vi "L298N_Controller.vi"(8 "Error In":errorcluster caption="Entrée d'erreur", 10 "Action_Moteur":T9, 11 "Cluster":T1) -> (0 "Error Out":errorcluster caption="Sortie d'erreur")   [LabVIEW 2019]
uses:
  L298N_Action_Enum.ctl
  L298N_Ref_Type.ctl
  <vilib>/myRIO/Instrument Drivers/Onboard IO/DIO/typedefs/DIO Reference.ctl
  <vilib>/myRIO/Common/Instrument Driver Framework/Utilities/typedefs/myRIO Generic Hardware Reference.ctl
  <vilib>/myRIO/Common/Instrument Driver Framework/Utilities/typedefs/Hardware Version Enum.ctl
  <vilib>/myRIO/Common/Instrument Driver Framework/Utilities/typedefs/myRIO v1.0 Reference.ctl
  <vilib>/myRIO/Common/Instrument Driver Framework/Utilities/typedefs/Generic FPGA Reference.ctl
  <vilib>/myRIO/Common/Instrument Driver Framework/myRIO v1.0/DIO/typedefs/DIO Channels List.ctl
  <vilib>/myRIO/Common/Instrument Driver Framework/myRIO v1.0/DIO/typedefs/DIO Channels Enum.ctl
  <vilib>/Utility/error.llb/Error Cluster From Error Code.vi
  <vilib>/myRIO/Common/Instrument Driver Framework/myRIO v1.0/DIO/vis/myRIO v1.0 Write DIO.vi
  <vilib>/myRIO/Instrument Drivers/Onboard IO/DIO/DIO.lvlib
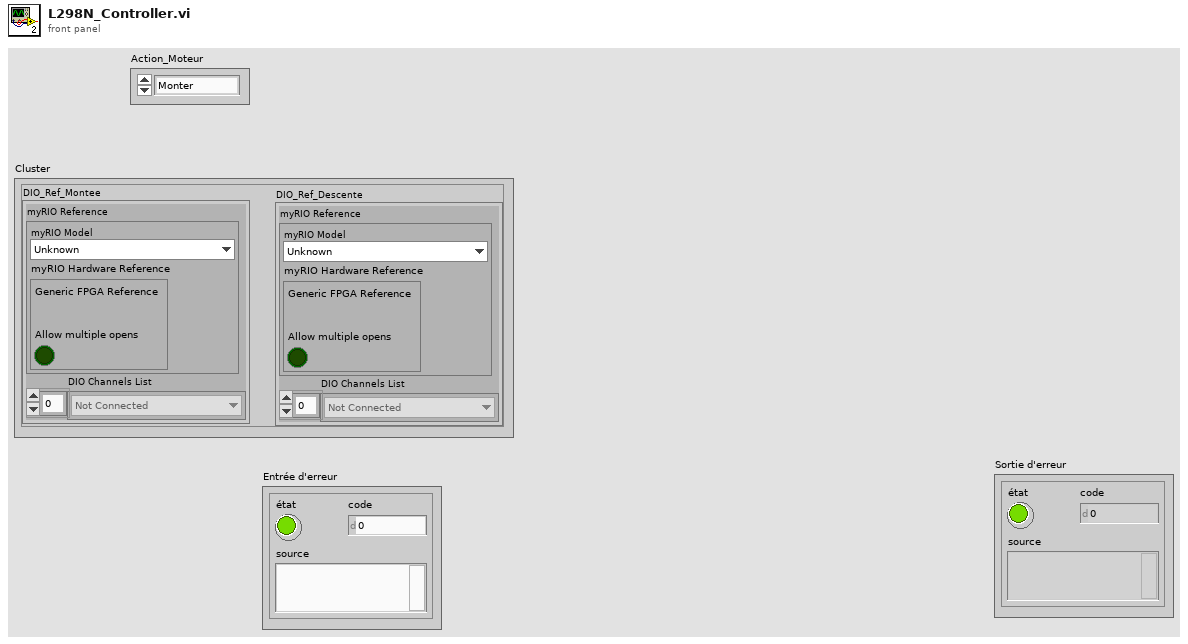
[diagram p1: front panel]
types:
  T1 = typedef "L298N_Ref_Type.ctl" = cluster{"DIO_Ref_Montee":T2, "DIO_Ref_Descente":T2}
  T2 = typedef "DIO.lvlib/DIO Reference.ctl" = cluster{"myRIO Reference":T3, "DIO Channels List":T7}
  T3 = typedef "myRIO Generic Hardware Reference.ctl" = cluster{"myRIO Model":T4, "myRIO Hardware Reference":T5}
  T4 = typedef "Hardware Version Enum.ctl" = enum16{"Unknown", "myRIO-1900", "myRIO-1950", "roboRIO", "NI ELVIS RIO CM", "ELVIS III"}
  T5 = typedef "myRIO v1.0 Reference.ctl" = cluster{"Generic FPGA Reference":T6, "Allow multiple opens":bool}
  T6 = typedef "Generic FPGA Reference.ctl" = refnum<k20>
  T7 = typedef "DIO Channels List.ctl" = T8[]
  T8 = typedef "DIO Channels Enum.ctl" = enum16{"Not Connected", "C/DIO0", "C/DIO1", "C/DIO2", "C/DIO3", "C/DIO4", "C/DIO5", "C/DIO6", "C/DIO7", "A/DIO0", "A/DIO1", "A/DIO2", "A/DIO3", "A/DIO4", "A/DIO5", "A/DIO6", "A/DIO7", "A/DIO8", "A/DIO9", "A/DIO10", "A/DIO11", "A/DIO12", "A/DIO13", "A/DIO14", "A/DIO15", "A/DIO16", "A/DIO17", "A/DIO18", "A/DIO19", "B/DIO0", "B/DIO1", "B/DIO2", "B/DIO3", "B/DIO4", "B/DIO5", "B/DIO6", "B/DIO7", "B/DIO8", "B/DIO9", "B/DIO10", "B/DIO11", "B/DIO12", "B/DIO13", "B/DIO14", "B/DIO15", "B/DIO16", "B/DIO17", "B/DIO18", "B/DIO19", "LED0", "LED1", "LED2", "LED3", "Button0", "DIO/DIO0", "DIO/DIO1", "DIO/DIO2", "DIO/DIO3", "DIO/DIO4", "DIO/DIO5", "DIO/DIO6", "DIO/DIO7", "DIO/DIO8", "DIO/DIO9", "SPI/CS0", "SPI/CS1", "SPI/CS2", "SPI/CS3", "LED RADIO (Green)", "LED RADIO (Red)", "LED COMM (Green)", "LED COMM (Red)", "LED MODE (Green)", "LED MODE (Red)"}
  T9 = typedef "L298N_Action_Enum.ctl" = enum16{"Monter", "Descendre", "Arreter"}
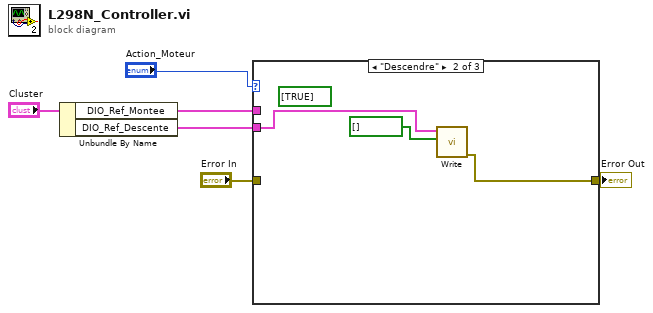
[diagram p0: block diagram]
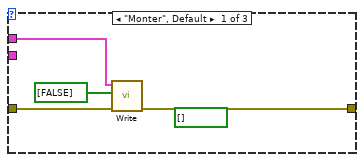
[diagram p2: hidden frame]
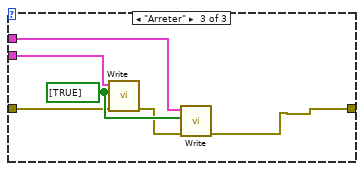
[diagram p3: hidden frame]
diagram:
  n1 = Unbundle By Name("Cluster") -> ("DIO_Ref_Montee"=w3:T2, "DIO_Ref_Descente"=w2:T2)
  n2 = case shown="\"Descendre\"" "Action_Moteur" {
    tunnel: w2 -> [_ w13 w19]
    tunnel: w3 -> [w8 _ w18]
    tunnel: "Error In" -> [w9 _ w16]
    tunnel: [w7 w11 w14] -> w5
    frame "Monter", Default {
      (unwired) bool[] [] ("Values")
      n3 = call <vilib>:"Write.vi"("error in (no error)"=w9, "Values"=bool[] [FALSE], "DIO Ref In"=w8) -> ("error out"=w7:errorcluster)  [unwired: 6 in, 1 out]
    }
    frame "Descendre" {
      (unwired) bool[] [TRUE] ("Values")
      n4 = call <vilib>:"Write.vi"("Values"=bool[] [], "DIO Ref In"=w13) -> ("error out"=w11:errorcluster)  [unwired: 7 in, 1 out]
    }
    frame "Arreter" {
      w17 = bool[] [TRUE] ("Values")
      n5 = call <vilib>:"Write.vi"("error in (no error)"=w16, "Values"=w17, "DIO Ref In"=w19) -> ("error out"=w15:errorcluster)  [unwired: 6 in, 1 out]
      n6 = call <vilib>:"Write.vi"("error in (no error)"=w15, "Values"=w17, "DIO Ref In"=w18) -> ("error out"=w14:errorcluster)  [unwired: 6 in, 1 out]
    }
  }
  "Error Out" <- w5
